vi "自定义项目符号.vi"() -> ()   [LabVIEW 2012, in "Tree Tools.lvlib"]
uses:
  Tree Tools.lvlib
  Core Class/Tree Class/Tree Class.lvclass
  Core Class/Tree Tag Class/Tree Tag Class.lvclass
  <userlib>/_OpenG.lib/file/file.llb/Strip Path Extension - String__ogtk.vi
  <userlib>/_OpenG.lib/file/file.llb/Build Path - Traditional__ogtk.vi
panel:
  in  "Quit":bool
  out "Data":variant
  in  "YourClusterName":T1
  in  "Tree":string(tree)
  # "1- Modify the above cluster at will\n2- Then run the VI."
  # "3- Select any item and to extract the value in \"Data\" variant field.\n4- Click on the glyphs to toggle them."
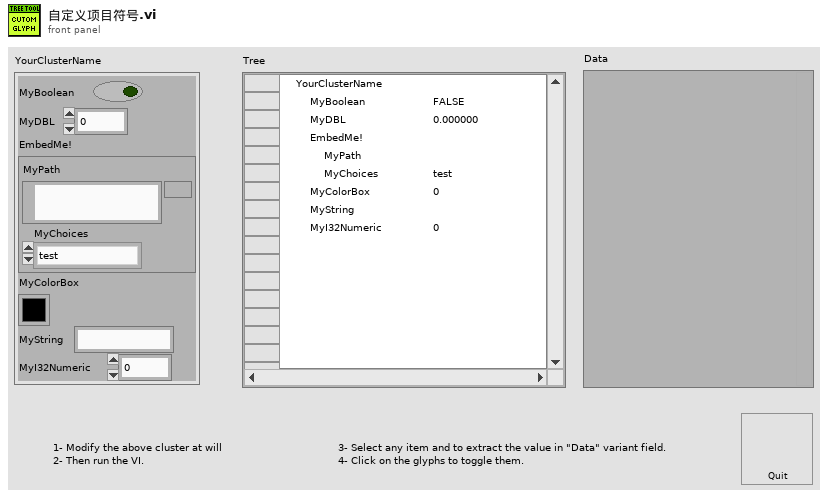
[diagram p1: front panel]
types:
  T1 = cluster{"MyBoolean":bool, "MyDBL":dbl, "EmbedMe!":cluster{"MyPath":path, "MyChoices":enum16{"test", "test1", "test3", "test5"}}, "MyColorBox":u32, "MyString":string, "MyI32Numeric":i32}
  T2 = typedef "imagedata.ctl" = cluster{"image type":i32, "image depth":i32, "image":u8[], "mask":u8[], "colors":u32[], "Rectangle":cluster{"left":i16, "top":i16, "right":i16, "bottom":i16}}
  T3 = cluster{"Hierarchy Lines":enum32{"Visible", "Invisible", "OS Default"}, "Symbols":bool, "Column Headers":bool, "Row Headers":bool, "Horizontal Lines":bool, "Vertical Lines":bool}
  T4 = typedef "LVPoint32TypeDef.ctl" = cluster{"Horizontal":i32, "Vertical":i32}
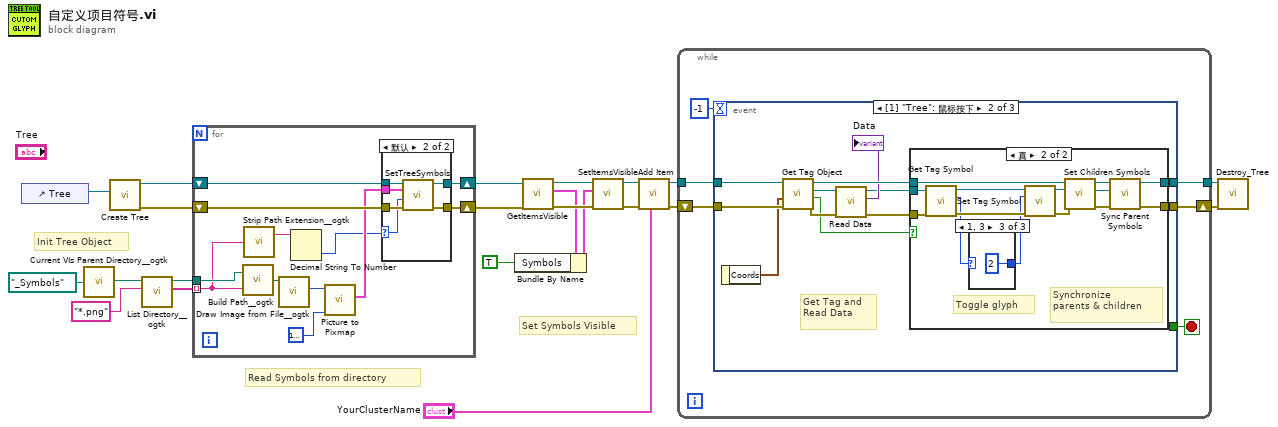
[diagram p0: block diagram]
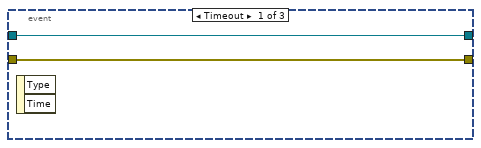
[diagram p3: hidden frame]
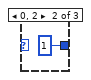
[diagram p6: hidden frame]
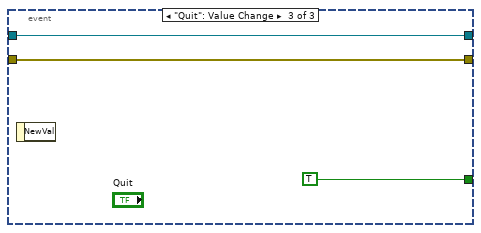
[diagram p7: hidden frame]
diagram:
  # "Init Tree Object"
  # "Read Symbols from directory"
  # "Set Symbols Visible"
  n1 = control-ref of="Tree"() -> (w9:refnum<vi>)
  n2 = call <userlib>:"Current VIs Parent Directory__ogtk.vi"("Relative path (.)"=path "_Symbols") -> ("Parent Directory (+ Relative)"=w15:path)  [unwired: 4 in]
  n3 = call "Create Tree.vi"("Tree Refnum"=w9) -> ("error out"=w7:errorcluster, "Tree_LVOOP out"=w8:refnum<class "Tree Class.lvclass">)  [unwired: 9 in]
  n4 = call <userlib>:"List Directory__ogtk.vi"("pattern"="*.png", "directory path"=w15) -> ("file names"=w13:string[], "dup directory path"=w10:path)  [unwired: 2 in, 2 out]
  n5 = for {
    tunnel: w13 -> [w23] mode=indexing
    shift-right: [w33] -> w12
    shift-left: w8 -> [w34]
    shift-right: [w32] -> w11
    shift-left: w7 -> [w31]
    tunnel: w10 -> [w27]
    n6 = call-poly <userlib>:"Build Path__ogtk.vi"("name or relative path"=w23, "base path"=w27) -> ("appended path"=w28:path)
    n7 = call-poly <userlib>:"Strip Path Extension__ogtk.vi"("path"=w23) -> ("root"=w26:string)  [unwired: 1 out]
    n8 = call <userlib>:"Draw Image from File__ogtk.vi"("path to image file"=w28) -> ("new picture"=w30:picture)  [unwired: 7 in, 3 out]
    n9 = Decimal String To Number(string=w26) -> (number=w25:i32)  [unwired: 3 out]
    n10 = call <vilib>:"Picture to Pixmap.vi"("Background Color"=u32 16777216, "picture"=w30) -> ("image data"=w29:T2)  [unwired: 2 in, 7 out]
    n11 = case shown="默认" w25 {
      selector: w25 -> [_ w37]
      tunnel: w34 -> [w36 w42]
      tunnel: [w36 w41] -> w33
      tunnel: [w35 w40] -> w32
      tunnel: w31 -> [w35 w39]
      tunnel: w29 -> [_ w38]
      frame ..0 {
      }
      frame Default {
        n12 = call-dynamic "SetTreeSymbols.vi"("error in (no error)"=w39, "Index"=w37, "Image"=w38, "Tree_LVOOP in"=w42) -> ("error out"=w40:errorcluster, "Tree_LVOOP out"=w41:refnum<class "Tree Class.lvclass">)  [unwired: 6 in]
      }
    }
  }
  n13 = call-dynamic "GetItemsVisible.vi"("error in (no error)"=w11, "Tree_LVOOP in"=w12) -> ("error out"=w19:errorcluster, "Visibility Cluster"=w18:T3, "Tree_LVOOP out"=w20:refnum<class "Tree Class.lvclass">)  [unwired: 7 in]
  n14 = Bundle By Name(cluster=w18, "Symbols"=TRUE) -> (w1:T3)
  n15 = call-dynamic "SetItemsVisible.vi"("error in (no error)"=w19, "Visibility Cluster"=w1, "Tree_LVOOP in"=w20) -> ("error out"=w3:errorcluster, "Tree_LVOOP out"=w6:refnum<class "Tree Class.lvclass">)  [unwired: 7 in]
  n16 = call-dynamic "Add Item.vi"("Data"="YourClusterName", "error in (no error)"=w3, "Tree_LVOOP in"=w6) -> ("error out"=w2:errorcluster, "Tree_LVOOP out"=w5:refnum<class "Tree Class.lvclass">)  [unwired: 6 in, 1 out]
  n17 = while {
    tunnel: w5 -> [w47]
    tunnel: [w46] -> w22
    shift-right: [w43] -> w21
    shift-left: w2 -> [w44]
    stop <- w45 stop-if-true
    n18 = event shown="[1] \"Tree\": 鼠标按下" {
      selector: _ -> [_ _ _]
      dyn-events: _ -> [_ _ _]
      timeout: -1 -> [_ _ _]
      tunnel: w47 -> [w50 w62 w83]
      tunnel: [w50 w57 w83] -> w46
      tunnel: [_ _ TRUE ("Delete Tree Items? (F)")] -> w45
      tunnel: w44 -> [w49 w61 w81]
      tunnel: [w49 w58 w81] -> w43
      event Timeout {
        n19 = event-data() -> ()  [unwired: 3 out]
      }
      event "Tree": Mouse Down {
        # "Get Tag and\nRead Data"
        n20 = event-data() -> ("Coords"=w60:T4)  [unwired: 1 out]
        n21 = call-dynamic "Get Tag Object.vi"("error in (no error)"=w61, "Coords (if tag empty)"=w60, "Tree_LVOOP in"=w62) -> ("error out"=w53:errorcluster, "InGlyph"=w51:bool, "Tag"=w56:refnum<class "Tree Tag Class.lvclass">, "Tree_LVOOP out"=w59:refnum<class "Tree Class.lvclass">)  [unwired: 5 in]
        n22 = call-dynamic "Read Data.vi"("error in (no error)"=w53, "Tag_LVOOP.lvclass in"=w56) -> ("error out"=w52:errorcluster, "Data"=→"Data":variant, "Tag_LVOOP.lvclass out"=w54:refnum<class "Tree Tag Class.lvclass">)  [unwired: 7 in]
        n23 = case shown="真" w51 {
          tunnel: w59 -> [w64 w73]
          tunnel: [w63 w72] -> w58
          tunnel: [w64 w70] -> w57
          tunnel: w54 -> [_ w66]
          tunnel: w52 -> [w63 w65]
          frame False {
          }
          frame True {
            # "Synchronize\nparents & children"
            # "Toggle glyph"
            n24 = call-dynamic "Get Tag Symbol.vi"("error in (no error)"=w65, "Tag_LVOOP in"=w66) -> ("error out"=w76:errorcluster, "Symbol Index"=w75:i32, "Tag_LVOOP out"=w77:refnum<class "Tree Tag Class.lvclass">)  [unwired: 7 in]
            n25 = case shown="1, 3" w75 {
              selector: w75 -> [w78 _ _]
              tunnel: [w78 1 ("Symbol Index") 2 ("Symbol Index")] -> w74
              frame Default {
              }
              frame 0, 2 {
              }
              frame 1, 3 {
              }
            }
            n26 = call-dynamic "Set Tag Symbol.vi"("error in (no error)"=w76, "Symbol Index"=w74, "Tag_LVOOP in"=w77) -> ("error out"=w67:errorcluster, "Tag_LVOOP out"=w68:refnum<class "Tree Tag Class.lvclass">)  [unwired: 7 in]
            n27 = call "Set Children Symbols.vi"("error in"=w67, "Parent tag"=w68, "Tree_LVOOP in"=w73) -> ("error out"=w69:errorcluster, "Tree_LVOOP out"=w71:refnum<class "Tree Class.lvclass">)  [unwired: 7 in]
            n28 = call-dynamic "Sync Parent Symbols.vi"("error in"=w69, "Child Tag_LVOOP"=w68, "Tree_LVOOP in"=w71) -> ("error out"=w72:errorcluster, "Tree_LVOOP out"=w70:refnum<class "Tree Class.lvclass">)  [unwired: 7 in]
          }
        }
      }
      event "Quit": Value Change {
        n29 = event-data() -> ()  [unwired: 2 out]
      }
    }
  }
  n30 = call-dynamic "Destroy_Tree.vi"("error in (no error)"=w21, "Tree_LVOOP in"=w22) -> ()  [unwired: 9 in, 1 out]
